vi "get bolt check tags.vi"(11 "PLC boolean read Tags":T3={"AT glass position"={"Tag Name"="", "Network Path"="", "use opc"=FALSE, "DataSocket Reference"={"CWDSLib._DCWDataSocket"=refnum, "CWDSLib._DCWData"=refnum, "OnDataUpdated"=0, "OnStatusUpdated"=0}}, "AT shade position"={"Tag Name"="", "Network Path"="", "use opc"=FALSE, "DataSocket Reference"={"CWDSLib._DCWDataSocket"=refnum, "CWDSLib._DCWData"=refnum, "OnDataUpdated"=0, "OnStatusUpdated"=0}}, "AT in glass wand lower pos"={"Tag Name"="", "Network Path"="", "use opc"=FALSE, "DataSocket Reference"={"CWDSLib._DCWDataSocket"=refnum, "CWDSLib._DCWData"=refnum, "OnDataUpdated"=0, "OnStatusUpdated"=0}}, "AT in sunshad wand lower pos"={"Tag Name"="", "Network Path"="", "use opc"=FALSE, "DataSocket Reference"={"CWDSLib._DCWDataSocket"=refnum, "CWDSLib._DCWData"=refnum, "OnDataUpdated"=0, "OnStatusUpdated"=0}}, "AT in wand home pos"={"Tag Name"="", "Network Path"="", "use opc"=FALSE, "DataSocket Reference"={"CWDSLib._DCWDataSocket"=refnum, "CWDSLib._DCWData"=refnum, "OnDataUpdated"=0, "OnStatusUpdated"=0}}, "LVDT's Extended"={"Tag Name"="", "Network Path"="", "use opc"=FALSE, "DataSocket Reference"={"CWDSLib._DCWDataSocket"=refnum, "CWDSLib._DCWData"=refnum, "OnDataUpdated"=0, "OnStatusUpdated"=0}}, "motor foam present LH"={"Tag Name"="", "Network Path"="", "use opc"=FALSE, "DataSocket Reference"={"CWDSLib._DCWDataSocket"=refnum, "CWDSLib._DCWData"=refnum, "OnDataUpdated"=0, "OnStatusUpdated"=0}}, "motor foam present RH"={"Tag Name"="", "Network Path"="", "use opc"=FALSE, "DataSocket Reference"={"CWDSLib._DCWDataSocket"=refnum, "CWDSLib._DCWData"=refnum, "OnDataUpdated"=0, "OnStatusUpdated"=0}}, "audit gap hider present LH"={"Tag Name"="", "Network Path"="", "use opc"=FALSE, "DataSocket Reference"={"CWDSLib._DCWDataSocket"=refnum, "CWDSLib._DCWData"=refnum, "OnDataUpdated"=0, "OnStatusUpdated"=0}}, "audit gap hider present RH"={"Tag Name"="", "Network Path"="", "use opc"=FALSE, "DataSocket Reference"={"CWDSLib._DCWDataSocket"=refnum, "CWDSLib._DCWData"=refnum, "OnDataUpdated"=0, "OnStatusUpdated"=0}}, "FB light block present"={"Tag Name"="", "Network Path"="", "use opc"=FALSE, "DataSocket Reference"={"CWDSLib._DCWDataSocket"=refnum, "CWDSLib._DCWData"=refnum, "OnDataUpdated"=0, "OnStatusUpdated"=0}}, "bolt check 1"={"Tag Name"="", "Network Path"="", "use opc"=FALSE, "DataSocket Reference"={"CWDSLib._DCWDataSocket"=refnum, "CWDSLib._DCWData"=refnum, "OnDataUpdated"=0, "OnStatusUpdated"=0}}, "bolt check 2"={"Tag Name"="", "Network Path"="", "use opc"=FALSE, "DataSocket Reference"={"CWDSLib._DCWDataSocket"=refnum, "CWDSLib._DCWData"=refnum, "OnDataUpdated"=0, "OnStatusUpdated"=0}}, "bolt check 3"={"Tag Name"="", "Network Path"="", "use opc"=FALSE, "DataSocket Reference"={"CWDSLib._DCWDataSocket"=refnum, "CWDSLib._DCWData"=refnum, "OnDataUpdated"=0, "OnStatusUpdated"=0}}, "bolt check 4"={"Tag Name"="", "Network Path"="", "use opc"=FALSE, "DataSocket Reference"={"CWDSLib._DCWDataSocket"=refnum, "CWDSLib._DCWData"=refnum, "OnDataUpdated"=0, "OnStatusUpdated"=0}}, "bolt check 5"={"Tag Name"="", "Network Path"="", "use opc"=FALSE, "DataSocket Reference"={"CWDSLib._DCWDataSocket"=refnum, "CWDSLib._DCWData"=refnum, "OnDataUpdated"=0, "OnStatusUpdated"=0}}, "bolt check 6"={"Tag Name"="", "Network Path"="", "use opc"=FALSE, "DataSocket Reference"={"CWDSLib._DCWDataSocket"=refnum, "CWDSLib._DCWData"=refnum, "OnDataUpdated"=0, "OnStatusUpdated"=0}}, "bolt check 7"={"Tag Name"="", "Network Path"="", "use opc"=FALSE, "DataSocket Reference"={"CWDSLib._DCWDataSocket"=refnum, "CWDSLib._DCWData"=refnum, "OnDataUpdated"=0, "OnStatusUpdated"=0}}, "bolt check 8"={"Tag Name"="", "Network Path"="", "use opc"=FALSE, "DataSocket Reference"={"CWDSLib._DCWDataSocket"=refnum, "CWDSLib._DCWData"=refnum, "OnDataUpdated"=0, "OnStatusUpdated"=0}}, "bolt check 9"={"Tag Name"="", "Network Path"="", "use opc"=FALSE, "DataSocket Reference"={"CWDSLib._DCWDataSocket"=refnum, "CWDSLib._DCWData"=refnum, "OnDataUpdated"=0, "OnStatusUpdated"=0}}, "bolt check 10"={"Tag Name"="", "Network Path"="", "use opc"=FALSE, "DataSocket Reference"={"CWDSLib._DCWDataSocket"=refnum, "CWDSLib._DCWData"=refnum, "OnDataUpdated"=0, "OnStatusUpdated"=0}}, "bolt check 11"={"Tag Name"="", "Network Path"="", "use opc"=FALSE, "DataSocket Reference"={"CWDSLib._DCWDataSocket"=refnum, "CWDSLib._DCWData"=refnum, "OnDataUpdated"=0, "OnStatusUpdated"=0}}, "bolt check 12"={"Tag Name"="", "Network Path"="", "use opc"=FALSE, "DataSocket Reference"={"CWDSLib._DCWDataSocket"=refnum, "CWDSLib._DCWData"=refnum, "OnDataUpdated"=0, "OnStatusUpdated"=0}}, "bolt check 13"={"Tag Name"="", "Network Path"="", "use opc"=FALSE, "DataSocket Reference"={"CWDSLib._DCWDataSocket"=refnum, "CWDSLib._DCWData"=refnum, "OnDataUpdated"=0, "OnStatusUpdated"=0}}, "bolt check 14"={"Tag Name"="", "Network Path"="", "use opc"=FALSE, "DataSocket Reference"={"CWDSLib._DCWDataSocket"=refnum, "CWDSLib._DCWData"=refnum, "OnDataUpdated"=0, "OnStatusUpdated"=0}}, "bolt check 15"={"Tag Name"="", "Network Path"="", "use opc"=FALSE, "DataSocket Reference"={"CWDSLib._DCWDataSocket"=refnum, "CWDSLib._DCWData"=refnum, "OnDataUpdated"=0, "OnStatusUpdated"=0}}, "bolt check 16"={"Tag Name"="", "Network Path"="", "use opc"=FALSE, "DataSocket Reference"={"CWDSLib._DCWDataSocket"=refnum, "CWDSLib._DCWData"=refnum, "OnDataUpdated"=0, "OnStatusUpdated"=0}}, "bolt check 17"={"Tag Name"="", "Network Path"="", "use opc"=FALSE, "DataSocket Reference"={"CWDSLib._DCWDataSocket"=refnum, "CWDSLib._DCWData"=refnum, "OnDataUpdated"=0, "OnStatusUpdated"=0}}, "bolt check 18"={"Tag Name"="", "Network Path"="", "use opc"=FALSE, "DataSocket Reference"={"CWDSLib._DCWDataSocket"=refnum, "CWDSLib._DCWData"=refnum, "OnDataUpdated"=0, "OnStatusUpdated"=0}}, "bolt check 19"={"Tag Name"="", "Network Path"="", "use opc"=FALSE, "DataSocket Reference"={"CWDSLib._DCWDataSocket"=refnum, "CWDSLib._DCWData"=refnum, "OnDataUpdated"=0, "OnStatusUpdated"=0}}, "bolt check 20"={"Tag Name"="", "Network Path"="", "use opc"=FALSE, "DataSocket Reference"={"CWDSLib._DCWDataSocket"=refnum, "CWDSLib._DCWData"=refnum, "OnDataUpdated"=0, "OnStatusUpdated"=0}}, "bolt check 21"={"Tag Name"="", "Network Path"="", "use opc"=FALSE, "DataSocket Reference"={"CWDSLib._DCWDataSocket"=refnum, "CWDSLib._DCWData"=refnum, "OnDataUpdated"=0, "OnStatusUpdated"=0}}, "start"={"Tag Name"="S060.PXI.Signals.PlltData.SN", "Network Path"="172.15.51.1,1,0", "use opc"=FALSE, "DataSocket Reference"={"CWDSLib._DCWDataSocket"=refnum, "CWDSLib._DCWData"=refnum, "OnDataUpdated"=0, "OnStatusUpdated"=0}}, "abort"={"Tag Name"="S060.PXI.Signals.PlltData.SN", "Network Path"="172.15.51.1,1,0", "use opc"=FALSE, "DataSocket Reference"={"CWDSLib._DCWDataSocket"=refnum, "CWDSLib._DCWData"=refnum, "OnDataUpdated"=0, "OnStatusUpdated"=0}}, "LVDT's Retracted"={"Tag Name"="S060.PXI.Signals.PlltData.SN", "Network Path"="172.15.51.1,1,0", "use opc"=FALSE, "DataSocket Reference"={"CWDSLib._DCWDataSocket"=refnum, "CWDSLib._DCWData"=refnum, "OnDataUpdated"=0, "OnStatusUpdated"=0}}, "manual barcode print"={"Tag Name"="S060.PXI.Signals.PlltData.SN", "Network Path"="172.15.51.1,1,0", "use opc"=FALSE, "DataSocket Reference"={"CWDSLib._DCWDataSocket"=refnum, "CWDSLib._DCWData"=refnum, "OnDataUpdated"=0, "OnStatusUpdated"=0}}, "ss servo at open"={"Tag Name"="S060.PXI.Signals.PlltData.SN", "Network Path"="172.15.51.1,1,0", "use opc"=FALSE, "DataSocket Reference"={"CWDSLib._DCWDataSocket"=refnum, "CWDSLib._DCWData"=refnum, "OnDataUpdated"=0, "OnStatusUpdated"=0}}, "ss servo at close"={"Tag Name"="S060.PXI.Signals.PlltData.SN", "Network Path"="172.15.51.1,1,0", "use opc"=FALSE, "DataSocket Reference"={"CWDSLib._DCWDataSocket"=refnum, "CWDSLib._DCWData"=refnum, "OnDataUpdated"=0, "OnStatusUpdated"=0}}, "ss servo opening"={"Tag Name"="S060.PXI.Signals.PlltData.SN", "Network Path"="172.15.51.1,1,0", "use opc"=FALSE, "DataSocket Reference"={"CWDSLib._DCWDataSocket"=refnum, "CWDSLib._DCWData"=refnum, "OnDataUpdated"=0, "OnStatusUpdated"=0}}, "ss servo closing"={"Tag Name"="S060.PXI.Signals.PlltData.SN", "Network Path"="172.15.51.1,1,0", "use opc"=FALSE, "DataSocket Reference"={"CWDSLib._DCWDataSocket"=refnum, "CWDSLib._DCWData"=refnum, "OnDataUpdated"=0, "OnStatusUpdated"=0}}, "control slide at home"={"Tag Name"="S060.PXI.Signals.PlltData.SN", "Network Path"="172.15.51.1,1,0", "use opc"=FALSE, "DataSocket Reference"={"CWDSLib._DCWDataSocket"=refnum, "CWDSLib._DCWData"=refnum, "OnDataUpdated"=0, "OnStatusUpdated"=0}}, "control slide left good"={"Tag Name"="S060.PXI.Signals.PlltData.SN", "Network Path"="172.15.51.1,1,0", "use opc"=FALSE, "DataSocket Reference"={"CWDSLib._DCWDataSocket"=refnum, "CWDSLib._DCWData"=refnum, "OnDataUpdated"=0, "OnStatusUpdated"=0}}, "control slide left over stroke"={"Tag Name"="S060.PXI.Signals.PlltData.SN", "Network Path"="172.15.51.1,1,0", "use opc"=FALSE, "DataSocket Reference"={"CWDSLib._DCWDataSocket"=refnum, "CWDSLib._DCWData"=refnum, "OnDataUpdated"=0, "OnStatusUpdated"=0}}, "control slide right good"={"Tag Name"="S060.PXI.Signals.PlltData.SN", "Network Path"="172.15.51.1,1,0", "use opc"=FALSE, "DataSocket Reference"={"CWDSLib._DCWDataSocket"=refnum, "CWDSLib._DCWData"=refnum, "OnDataUpdated"=0, "OnStatusUpdated"=0}}, "control slide right over stroke"={"Tag Name"="S060.PXI.Signals.PlltData.SN", "Network Path"="172.15.51.1,1,0", "use opc"=FALSE, "DataSocket Reference"={"CWDSLib._DCWDataSocket"=refnum, "CWDSLib._DCWData"=refnum, "OnDataUpdated"=0, "OnStatusUpdated"=0}}, "wind deflector high speed pos"={"Tag Name"="S060.PXI.Signals.PlltData.SN", "Network Path"="172.15.51.1,1,0", "use opc"=FALSE, "DataSocket Reference"={"CWDSLib._DCWDataSocket"=refnum, "CWDSLib._DCWData"=refnum, "OnDataUpdated"=0, "OnStatusUpdated"=0}}, "wind deflector low speed pos"={"Tag Name"="S060.PXI.Signals.PlltData.SN", "Network Path"="172.15.51.1,1,0", "use opc"=FALSE, "DataSocket Reference"={"CWDSLib._DCWDataSocket"=refnum, "CWDSLib._DCWData"=refnum, "OnDataUpdated"=0, "OnStatusUpdated"=0}}, "AT VentPMACatHome"={"Tag Name"="S060.PXI.Signals.PlltData.SN", "Network Path"="172.15.51.1,1,0", "use opc"=FALSE, "DataSocket Reference"={"CWDSLib._DCWDataSocket"=refnum, "CWDSLib._DCWData"=refnum, "OnDataUpdated"=0, "OnStatusUpdated"=0}}, "AT VentPMACisExtend"={"Tag Name"="S060.PXI.Signals.PlltData.SN", "Network Path"="172.15.51.1,1,0", "use opc"=FALSE, "DataSocket Reference"={"CWDSLib._DCWDataSocket"=refnum, "CWDSLib._DCWData"=refnum, "OnDataUpdated"=0, "OnStatusUpdated"=0}}, "SS Barcode Scanner Bypassed"={"Tag Name"="S060.PXI.Signals.PlltData.SN", "Network Path"="172.15.51.1,1,0", "use opc"=FALSE, "DataSocket Reference"={"CWDSLib._DCWDataSocket"=refnum, "CWDSLib._DCWData"=refnum, "OnDataUpdated"=0, "OnStatusUpdated"=0}}, "Check Frame Barcode"={"Tag Name"="S060.PXI.Signals.PlltData.SN", "Network Path"="172.15.51.1,1,0", "use opc"=FALSE, "DataSocket Reference"={"CWDSLib._DCWDataSocket"=refnum, "CWDSLib._DCWData"=refnum, "OnDataUpdated"=0, "OnStatusUpdated"=0}}, "iGPS Pass 0"={"Tag Name"="S060.PXI.Signals.PlltData.SN", "Network Path"="172.15.51.1,1,0", "use opc"=FALSE, "DataSocket Reference"={"CWDSLib._DCWDataSocket"=refnum, "CWDSLib._DCWData"=refnum, "OnDataUpdated"=0, "OnStatusUpdated"=0}}, "iGPS Pass 1"={"Tag Name"="S060.PXI.Signals.PlltData.SN", "Network Path"="172.15.51.1,1,0", "use opc"=FALSE, "DataSocket Reference"={"CWDSLib._DCWDataSocket"=refnum, "CWDSLib._DCWData"=refnum, "OnDataUpdated"=0, "OnStatusUpdated"=0}}, "iGPS Pass 2"={"Tag Name"="S060.PXI.Signals.PlltData.SN", "Network Path"="172.15.51.1,1,0", "use opc"=FALSE, "DataSocket Reference"={"CWDSLib._DCWDataSocket"=refnum, "CWDSLib._DCWData"=refnum, "OnDataUpdated"=0, "OnStatusUpdated"=0}}, "iGPS Pass 3"={"Tag Name"="S060.PXI.Signals.PlltData.SN", "Network Path"="172.15.51.1,1,0", "use opc"=FALSE, "DataSocket Reference"={"CWDSLib._DCWDataSocket"=refnum, "CWDSLib._DCWData"=refnum, "OnDataUpdated"=0, "OnStatusUpdated"=0}}, "iGPS Pass 4"={"Tag Name"="S060.PXI.Signals.PlltData.SN", "Network Path"="172.15.51.1,1,0", "use opc"=FALSE, "DataSocket Reference"={"CWDSLib._DCWDataSocket"=refnum, "CWDSLib._DCWData"=refnum, "OnDataUpdated"=0, "OnStatusUpdated"=0}}, "iGPS Pass 5"={"Tag Name"="S060.PXI.Signals.PlltData.SN", "Network Path"="172.15.51.1,1,0", "use opc"=FALSE, "DataSocket Reference"={"CWDSLib._DCWDataSocket"=refnum, "CWDSLib._DCWData"=refnum, "OnDataUpdated"=0, "OnStatusUpdated"=0}}, "iGPS Pass 6"={"Tag Name"="S060.PXI.Signals.PlltData.SN", "Network Path"="172.15.51.1,1,0", "use opc"=FALSE, "DataSocket Reference"={"CWDSLib._DCWDataSocket"=refnum, "CWDSLib._DCWData"=refnum, "OnDataUpdated"=0, "OnStatusUpdated"=0}}, "iGPS Pass 7"={"Tag Name"="S060.PXI.Signals.PlltData.SN", "Network Path"="172.15.51.1,1,0", "use opc"=FALSE, "DataSocket Reference"={"CWDSLib._DCWDataSocket"=refnum, "CWDSLib._DCWData"=refnum, "OnDataUpdated"=0, "OnStatusUpdated"=0}}, "iGPS Pass 8"={"Tag Name"="S060.PXI.Signals.PlltData.SN", "Network Path"="172.15.51.1,1,0", "use opc"=FALSE, "DataSocket Reference"={"CWDSLib._DCWDataSocket"=refnum, "CWDSLib._DCWData"=refnum, "OnDataUpdated"=0, "OnStatusUpdated"=0}}, "iGPS Pass 9"={"Tag Name"="S060.PXI.Signals.PlltData.SN", "Network Path"="172.15.51.1,1,0", "use opc"=FALSE, "DataSocket Reference"={"CWDSLib._DCWDataSocket"=refnum, "CWDSLib._DCWData"=refnum, "OnDataUpdated"=0, "OnStatusUpdated"=0}}, "Z LVDTs Extended"={"Tag Name"="S060.PXI.Signals.PlltData.SN", "Network Path"="172.15.51.1,1,0", "use opc"=FALSE, "DataSocket Reference"={"CWDSLib._DCWDataSocket"=refnum, "CWDSLib._DCWData"=refnum, "OnDataUpdated"=0, "OnStatusUpdated"=0}}, "NVH Operator Pass"={"Tag Name"="S060.PXI.Signals.PlltData.SN", "Network Path"="172.15.51.1,1,0", "use opc"=FALSE, "DataSocket Reference"={"CWDSLib._DCWDataSocket"=refnum, "CWDSLib._DCWData"=refnum, "OnDataUpdated"=0, "OnStatusUpdated"=0}}, "NVH Operator Fail"={"Tag Name"="S060.PXI.Signals.PlltData.SN", "Network Path"="172.15.51.1,1,0", "use opc"=FALSE, "DataSocket Reference"={"CWDSLib._DCWDataSocket"=refnum, "CWDSLib._DCWData"=refnum, "OnDataUpdated"=0, "OnStatusUpdated"=0}}, "NVH Operator Express Glass Open"={"Tag Name"="S060.PXI.Signals.PlltData.SN", "Network Path"="172.15.51.1,1,0", "use opc"=FALSE, "DataSocket Reference"={"CWDSLib._DCWDataSocket"=refnum, "CWDSLib._DCWData"=refnum, "OnDataUpdated"=0, "OnStatusUpdated"=0}}, "NVH Operator Express Glass Close"={"Tag Name"="S060.PXI.Signals.PlltData.SN", "Network Path"="172.15.51.1,1,0", "use opc"=FALSE, "DataSocket Reference"={"CWDSLib._DCWDataSocket"=refnum, "CWDSLib._DCWData"=refnum, "OnDataUpdated"=0, "OnStatusUpdated"=0}}, "NVH Operator Express Rollo Open01"={"Tag Name"="S060.PXI.Signals.PlltData.SN", "Network Path"="172.15.51.1,1,0", "use opc"=FALSE, "DataSocket Reference"={"CWDSLib._DCWDataSocket"=refnum, "CWDSLib._DCWData"=refnum, "OnDataUpdated"=0, "OnStatusUpdated"=0}}, "NVH Operator Express Rollo Close01"={"Tag Name"="S060.PXI.Signals.PlltData.SN", "Network Path"="172.15.51.1,1,0", "use opc"=FALSE, "DataSocket Reference"={"CWDSLib._DCWDataSocket"=refnum, "CWDSLib._DCWData"=refnum, "OnDataUpdated"=0, "OnStatusUpdated"=0}}, "NVH Operator Express Rollo Open02"={"Tag Name"="S060.PXI.Signals.PlltData.SN", "Network Path"="172.15.51.1,1,0", "use opc"=FALSE, "DataSocket Reference"={"CWDSLib._DCWDataSocket"=refnum, "CWDSLib._DCWData"=refnum, "OnDataUpdated"=0, "OnStatusUpdated"=0}}, "NVH Operator Express Rollo Close02"={"Tag Name"="S060.PXI.Signals.PlltData.SN", "Network Path"="172.15.51.1,1,0", "use opc"=FALSE, "DataSocket Reference"={"CWDSLib._DCWDataSocket"=refnum, "CWDSLib._DCWData"=refnum, "OnDataUpdated"=0, "OnStatusUpdated"=0}}, "NVH Operator Vent Open Noise"={"Tag Name"="S060.PXI.Signals.PlltData.SN", "Network Path"="172.15.51.1,1,0", "use opc"=FALSE, "DataSocket Reference"={"CWDSLib._DCWDataSocket"=refnum, "CWDSLib._DCWData"=refnum, "OnDataUpdated"=0, "OnStatusUpdated"=0}}, "NVH Operator Vent Close Noise"={"Tag Name"="S060.PXI.Signals.PlltData.SN", "Network Path"="172.15.51.1,1,0", "use opc"=FALSE, "DataSocket Reference"={"CWDSLib._DCWDataSocket"=refnum, "CWDSLib._DCWData"=refnum, "OnDataUpdated"=0, "OnStatusUpdated"=0}}, "NVH Operator Sunshade Open Noise"={"Tag Name"="S060.PXI.Signals.PlltData.SN", "Network Path"="172.15.51.1,1,0", "use opc"=FALSE, "DataSocket Reference"={"CWDSLib._DCWDataSocket"=refnum, "CWDSLib._DCWData"=refnum, "OnDataUpdated"=0, "OnStatusUpdated"=0}}, "NVH Operator Sunshade Close Noise"={"Tag Name"="S060.PXI.Signals.PlltData.SN", "Network Path"="172.15.51.1,1,0", "use opc"=FALSE, "DataSocket Reference"={"CWDSLib._DCWDataSocket"=refnum, "CWDSLib._DCWData"=refnum, "OnDataUpdated"=0, "OnStatusUpdated"=0}}, "NVH Operator Glass Open Noise"={"Tag Name"="S060.PXI.Signals.PlltData.SN", "Network Path"="172.15.51.1,1,0", "use opc"=FALSE, "DataSocket Reference"={"CWDSLib._DCWDataSocket"=refnum, "CWDSLib._DCWData"=refnum, "OnDataUpdated"=0, "OnStatusUpdated"=0}}, "NVH Operator Glass Close Noise"={"Tag Name"="S060.PXI.Signals.PlltData.SN", "Network Path"="172.15.51.1,1,0", "use opc"=FALSE, "DataSocket Reference"={"CWDSLib._DCWDataSocket"=refnum, "CWDSLib._DCWData"=refnum, "OnDataUpdated"=0, "OnStatusUpdated"=0}}, "NVH Operator Finish"={"Tag Name"="S060.PXI.Signals.PlltData.SN", "Network Path"="172.15.51.1,1,0", "use opc"=FALSE, "DataSocket Reference"={"CWDSLib._DCWDataSocket"=refnum, "CWDSLib._DCWData"=refnum, "OnDataUpdated"=0, "OnStatusUpdated"=0}}, "NVH Operator Check"={"Tag Name"="S060.PXI.Signals.PlltData.SN", "Network Path"="172.15.51.1,1,0", "use opc"=FALSE, "DataSocket Reference"={"CWDSLib._DCWDataSocket"=refnum, "CWDSLib._DCWData"=refnum, "OnDataUpdated"=0, "OnStatusUpdated"=0}}, "AT shade 02 position"={"Tag Name"="S060.PXI.Signals.PlltData.SN", "Network Path"="172.15.51.1,1,0", "use opc"=FALSE, "DataSocket Reference"={"CWDSLib._DCWDataSocket"=refnum, "CWDSLib._DCWData"=refnum, "OnDataUpdated"=0, "OnStatusUpdated"=0}}, "AT in sunshad 02 wand up pos"={"Tag Name"="S060.PXI.Signals.PlltData.SN", "Network Path"="172.15.51.1,1,0", "use opc"=FALSE, "DataSocket Reference"={"CWDSLib._DCWDataSocket"=refnum, "CWDSLib._DCWData"=refnum, "OnDataUpdated"=0, "OnStatusUpdated"=0}}, "AT in wand 02 home pos"={"Tag Name"="S060.PXI.Signals.PlltData.SN", "Network Path"="172.15.51.1,1,0", "use opc"=FALSE, "DataSocket Reference"={"CWDSLib._DCWDataSocket"=refnum, "CWDSLib._DCWData"=refnum, "OnDataUpdated"=0, "OnStatusUpdated"=0}}, "windproof position"={"Tag Name"="S060.PXI.Signals.PlltData.SN", "Network Path"="172.15.51.1,1,0", "use opc"=FALSE, "DataSocket Reference"={"CWDSLib._DCWDataSocket"=refnum, "CWDSLib._DCWData"=refnum, "OnDataUpdated"=0, "OnStatusUpdated"=0}}, "NVH Operator Express Glass vent Open"={"Tag Name"="S060.PXI.Signals.PlltData.SN", "Network Path"="172.15.51.1,1,0", "use opc"=FALSE, "DataSocket Reference"={"CWDSLib._DCWDataSocket"=refnum, "CWDSLib._DCWData"=refnum, "OnDataUpdated"=0, "OnStatusUpdated"=0}}, "NVH Operator Express Glass Vent Close"={"Tag Name"="S060.PXI.Signals.PlltData.SN", "Network Path"="172.15.51.1,1,0", "use opc"=FALSE, "DataSocket Reference"={"CWDSLib._DCWDataSocket"=refnum, "CWDSLib._DCWData"=refnum, "OnDataUpdated"=0, "OnStatusUpdated"=0}}, "NVH Operator Re-do"={"Tag Name"="S060.PXI.Signals.PlltData.SN", "Network Path"="172.15.51.1,1,0", "use opc"=FALSE, "DataSocket Reference"={"CWDSLib._DCWDataSocket"=refnum, "CWDSLib._DCWData"=refnum, "OnDataUpdated"=0, "OnStatusUpdated"=0}}, "AT at vent ATS test pos"={"Tag Name"="S060.PXI.Signals.PlltData.SN", "Network Path"="172.15.51.1,1,0", "use opc"=FALSE, "DataSocket Reference"={"CWDSLib._DCWDataSocket"=refnum, "CWDSLib._DCWData"=refnum, "OnDataUpdated"=0, "OnStatusUpdated"=0}}, "AT at vent ATS Home pos"={"Tag Name"="S060.PXI.Signals.PlltData.SN", "Network Path"="172.15.51.1,1,0", "use opc"=FALSE, "DataSocket Reference"={"CWDSLib._DCWDataSocket"=refnum, "CWDSLib._DCWData"=refnum, "OnDataUpdated"=0, "OnStatusUpdated"=0}}, "Start Adjust LVDT"={"Tag Name"="S060.PXI.Signals.PlltData.SN", "Network Path"="172.15.51.1,1,0", "use opc"=FALSE, "DataSocket Reference"={"CWDSLib._DCWDataSocket"=refnum, "CWDSLib._DCWData"=refnum, "OnDataUpdated"=0, "OnStatusUpdated"=0}}, "Finish Adjust LVDT"={"Tag Name"="S060.PXI.Signals.PlltData.SN", "Network Path"="172.15.51.1,1,0", "use opc"=FALSE, "DataSocket Reference"={"CWDSLib._DCWDataSocket"=refnum, "CWDSLib._DCWData"=refnum, "OnDataUpdated"=0, "OnStatusUpdated"=0}}} {"Finish Adjust LVDT"."DataSocket Reference"."OnStatusUpdated" format="%.0x"; "Finish Adjust LVDT"."DataSocket Reference"."OnDataUpdated" format="%.0x"; "Start Adjust LVDT"."DataSocket Reference"."OnStatusUpdated" format="%.0x"; "Start Adjust LVDT"."DataSocket Reference"."OnDataUpdated" format="%.0x"; "AT at vent ATS Home pos"."DataSocket Reference"."OnStatusUpdated" format="%.0x"; "AT at vent ATS Home pos"."DataSocket Reference"."OnDataUpdated" format="%.0x"; "AT at vent ATS test pos"."DataSocket Reference"."OnStatusUpdated" format="%.0x"; "AT at vent ATS test pos"."DataSocket Reference"."OnDataUpdated" format="%.0x"; "NVH Operator Re-do"."DataSocket Reference"."OnStatusUpdated" format="%.0x"; "NVH Operator Re-do"."DataSocket Reference"."OnDataUpdated" format="%.0x"; "NVH Operator Express Glass Vent Close"."DataSocket Reference"."OnStatusUpdated" format="%.0x"; "NVH Operator Express Glass Vent Close"."DataSocket Reference"."OnDataUpdated" format="%.0x"; "NVH Operator Express Glass vent Open"."DataSocket Reference"."OnStatusUpdated" format="%.0x"; "NVH Operator Express Glass vent Open"."DataSocket Reference"."OnDataUpdated" format="%.0x"; "windproof position"."DataSocket Reference"."OnStatusUpdated" format="%.0x"; "windproof position"."DataSocket Reference"."OnDataUpdated" format="%.0x"; "AT in wand 02 home pos"."DataSocket Reference"."OnStatusUpdated" format="%.0x"; "AT in wand 02 home pos"."DataSocket Reference"."OnDataUpdated" format="%.0x"; "AT in sunshad 02 wand up pos"."DataSocket Reference"."OnStatusUpdated" format="%.0x"; "AT in sunshad 02 wand up pos"."DataSocket Reference"."OnDataUpdated" format="%.0x"; "AT shade 02 position"."DataSocket Reference"."OnStatusUpdated" format="%.0x"; "AT shade 02 position"."DataSocket Reference"."OnDataUpdated" format="%.0x"; "NVH Operator Check"."DataSocket Reference"."OnStatusUpdated" format="%.0x"; "NVH Operator Check"."DataSocket Reference"."OnDataUpdated" format="%.0x"; "NVH Operator Finish"."DataSocket Reference"."OnStatusUpdated" format="%.0x"; "NVH Operator Finish"."DataSocket Reference"."OnDataUpdated" format="%.0x"; "NVH Operator Glass Close Noise"."DataSocket Reference"."OnStatusUpdated" format="%.0x"; "NVH Operator Glass Close Noise"."DataSocket Reference"."OnDataUpdated" format="%.0x"; "NVH Operator Glass Open Noise"."DataSocket Reference"."OnStatusUpdated" format="%.0x"; "NVH Operator Glass Open Noise"."DataSocket Reference"."OnDataUpdated" format="%.0x"; "NVH Operator Sunshade Close Noise"."DataSocket Reference"."OnStatusUpdated" format="%.0x"; "NVH Operator Sunshade Close Noise"."DataSocket Reference"."OnDataUpdated" format="%.0x"; "NVH Operator Sunshade Open Noise"."DataSocket Reference"."OnStatusUpdated" format="%.0x"; "NVH Operator Sunshade Open Noise"."DataSocket Reference"."OnDataUpdated" format="%.0x"; "NVH Operator Vent Close Noise"."DataSocket Reference"."OnStatusUpdated" format="%.0x"; "NVH Operator Vent Close Noise"."DataSocket Reference"."OnDataUpdated" format="%.0x"; "NVH Operator Vent Open Noise"."DataSocket Reference"."OnStatusUpdated" format="%.0x"; "NVH Operator Vent Open Noise"."DataSocket Reference"."OnDataUpdated" format="%.0x"; "NVH Operator Express Rollo Close02"."DataSocket Reference"."OnStatusUpdated" format="%.0x"; "NVH Operator Express Rollo Close02"."DataSocket Reference"."OnDataUpdated" format="%.0x"; "NVH Operator Express Rollo Open02"."DataSocket Reference"."OnStatusUpdated" format="%.0x"; "NVH Operator Express Rollo Open02"."DataSocket Reference"."OnDataUpdated" format="%.0x"; "NVH Operator Express Rollo Close01"."DataSocket Reference"."OnStatusUpdated" format="%.0x"; "NVH Operator Express Rollo Close01"."DataSocket Reference"."OnDataUpdated" format="%.0x"; "NVH Operator Express Rollo Open01"."DataSocket Reference"."OnStatusUpdated" format="%.0x"; "NVH Operator Express Rollo Open01"."DataSocket Reference"."OnDataUpdated" format="%.0x"; "NVH Operator Express Glass Close"."DataSocket Reference"."OnStatusUpdated" format="%.0x"; "NVH Operator Express Glass Close"."DataSocket Reference"."OnDataUpdated" format="%.0x"; "NVH Operator Express Glass Open"."DataSocket Reference"."OnStatusUpdated" format="%.0x"; "NVH Operator Express Glass Open"."DataSocket Reference"."OnDataUpdated" format="%.0x"; "NVH Operator Fail"."DataSocket Reference"."OnStatusUpdated" format="%.0x"; "NVH Operator Fail"."DataSocket Reference"."OnDataUpdated" format="%.0x"; "NVH Operator Pass"."DataSocket Reference"."OnStatusUpdated" format="%.0x"; "NVH Operator Pass"."DataSocket Reference"."OnDataUpdated" format="%.0x"; "Z LVDTs Extended"."DataSocket Reference"."OnStatusUpdated" format="%.0x"; "Z LVDTs Extended"."DataSocket Reference"."OnDataUpdated" format="%.0x"; "iGPS Pass 9"."DataSocket Reference"."OnStatusUpdated" format="%.0x"; "iGPS Pass 9"."DataSocket Reference"."OnDataUpdated" format="%.0x"; "iGPS Pass 8"."DataSocket Reference"."OnStatusUpdated" format="%.0x"; "iGPS Pass 8"."DataSocket Reference"."OnDataUpdated" format="%.0x"; "iGPS Pass 7"."DataSocket Reference"."OnStatusUpdated" format="%.0x"; "iGPS Pass 7"."DataSocket Reference"."OnDataUpdated" format="%.0x"; "iGPS Pass 6"."DataSocket Reference"."OnStatusUpdated" format="%.0x"; "iGPS Pass 6"."DataSocket Reference"."OnDataUpdated" format="%.0x"; "iGPS Pass 5"."DataSocket Reference"."OnStatusUpdated" format="%.0x"; "iGPS Pass 5"."DataSocket Reference"."OnDataUpdated" format="%.0x"; "iGPS Pass 4"."DataSocket Reference"."OnStatusUpdated" format="%.0x"; "iGPS Pass 4"."DataSocket Reference"."OnDataUpdated" format="%.0x"; "iGPS Pass 3"."DataSocket Reference"."OnStatusUpdated" format="%.0x"; "iGPS Pass 3"."DataSocket Reference"."OnDataUpdated" format="%.0x"; "iGPS Pass 2"."DataSocket Reference"."OnStatusUpdated" format="%.0x"; "iGPS Pass 2"."DataSocket Reference"."OnDataUpdated" format="%.0x"; "iGPS Pass 1"."DataSocket Reference"."OnStatusUpdated" format="%.0x"; "iGPS Pass 1"."DataSocket Reference"."OnDataUpdated" format="%.0x"; "iGPS Pass 0"."DataSocket Reference"."OnStatusUpdated" format="%.0x"; "iGPS Pass 0"."DataSocket Reference"."OnDataUpdated" format="%.0x"; "Check Frame Barcode"."DataSocket Reference"."OnStatusUpdated" format="%.0x"; "Check Frame Barcode"."DataSocket Reference"."OnDataUpdated" format="%.0x"; "SS Barcode Scanner Bypassed"."DataSocket Reference"."OnStatusUpdated" format="%.0x"; "SS Barcode Scanner Bypassed"."DataSocket Reference"."OnDataUpdated" format="%.0x"; "AT VentPMACisExtend"."DataSocket Reference"."OnStatusUpdated" format="%.0x"; "AT VentPMACisExtend"."DataSocket Reference"."OnDataUpdated" format="%.0x"; "AT VentPMACatHome"."DataSocket Reference"."OnStatusUpdated" format="%.0x"; "AT VentPMACatHome"."DataSocket Reference"."OnDataUpdated" format="%.0x"; "wind deflector low speed pos"."DataSocket Reference"."OnStatusUpdated" format="%.0x"; "wind deflector low speed pos"."DataSocket Reference"."OnDataUpdated" format="%.0x"; "wind deflector high speed pos"."DataSocket Reference"."OnStatusUpdated" format="%.0x"; "wind deflector high speed pos"."DataSocket Reference"."OnDataUpdated" format="%.0x"; "control slide right over stroke"."DataSocket Reference"."OnStatusUpdated" format="%.0x"; "control slide right over stroke"."DataSocket Reference"."OnDataUpdated" format="%.0x"; "control slide right good"."DataSocket Reference"."OnStatusUpdated" format="%.0x"; "control slide right good"."DataSocket Reference"."OnDataUpdated" format="%.0x"; "control slide left over stroke"."DataSocket Reference"."OnStatusUpdated" format="%.0x"; "control slide left over stroke"."DataSocket Reference"."OnDataUpdated" format="%.0x"; "control slide left good"."DataSocket Reference"."OnStatusUpdated" format="%.0x"; "control slide left good"."DataSocket Reference"."OnDataUpdated" format="%.0x"; "control slide at home"."DataSocket Reference"."OnStatusUpdated" format="%.0x"; "control slide at home"."DataSocket Reference"."OnDataUpdated" format="%.0x"; "ss servo closing"."DataSocket Reference"."OnStatusUpdated" format="%.0x"; "ss servo closing"."DataSocket Reference"."OnDataUpdated" format="%.0x"; "ss servo opening"."DataSocket Reference"."OnStatusUpdated" format="%.0x"; "ss servo opening"."DataSocket Reference"."OnDataUpdated" format="%.0x"; "ss servo at close"."DataSocket Reference"."OnStatusUpdated" format="%.0x"; "ss servo at close"."DataSocket Reference"."OnDataUpdated" format="%.0x"; "ss servo at open"."DataSocket Reference"."OnStatusUpdated" format="%.0x"; "ss servo at open"."DataSocket Reference"."OnDataUpdated" format="%.0x"; "manual barcode print"."DataSocket Reference"."OnStatusUpdated" format="%.0x"; "manual barcode print"."DataSocket Reference"."OnDataUpdated" format="%.0x"; "LVDT's Retracted"."DataSocket Reference"."OnStatusUpdated" format="%.0x"; "LVDT's Retracted"."DataSocket Reference"."OnDataUpdated" format="%.0x"; "abort"."DataSocket Reference"."OnStatusUpdated" format="%.0x"; "abort"."DataSocket Reference"."OnDataUpdated" format="%.0x"; "start"."DataSocket Reference"."OnStatusUpdated" format="%.0x"; "start"."DataSocket Reference"."OnDataUpdated" format="%.0x"; "bolt check 21"."DataSocket Reference"."OnStatusUpdated" format="%.0x"; "bolt check 21"."DataSocket Reference"."OnDataUpdated" format="%.0x"; "bolt check 20"."DataSocket Reference"."OnStatusUpdated" format="%.0x"; "bolt check 20"."DataSocket Reference"."OnDataUpdated" format="%.0x"; "bolt check 19"."DataSocket Reference"."OnStatusUpdated" format="%.0x"; "bolt check 19"."DataSocket Reference"."OnDataUpdated" format="%.0x"; "bolt check 18"."DataSocket Reference"."OnStatusUpdated" format="%.0x"; "bolt check 18"."DataSocket Reference"."OnDataUpdated" format="%.0x"; "bolt check 17"."DataSocket Reference"."OnStatusUpdated" format="%.0x"; "bolt check 17"."DataSocket Reference"."OnDataUpdated" format="%.0x"; "bolt check 16"."DataSocket Reference"."OnStatusUpdated" format="%.0x"; "bolt check 16"."DataSocket Reference"."OnDataUpdated" format="%.0x"; "bolt check 15"."DataSocket Reference"."OnStatusUpdated" format="%.0x"; "bolt check 15"."DataSocket Reference"."OnDataUpdated" format="%.0x"; "bolt check 14"."DataSocket Reference"."OnStatusUpdated" format="%.0x"; "bolt check 14"."DataSocket Reference"."OnDataUpdated" format="%.0x"; "bolt check 13"."DataSocket Reference"."OnStatusUpdated" format="%.0x"; "bolt check 13"."DataSocket Reference"."OnDataUpdated" format="%.0x"; "bolt check 12"."DataSocket Reference"."OnStatusUpdated" format="%.0x"; "bolt check 12"."DataSocket Reference"."OnDataUpdated" format="%.0x"; "bolt check 11"."DataSocket Reference"."OnStatusUpdated" format="%.0x"; "bolt check 11"."DataSocket Reference"."OnDataUpdated" format="%.0x"; "bolt check 10"."DataSocket Reference"."OnStatusUpdated" format="%.0x"; "bolt check 10"."DataSocket Reference"."OnDataUpdated" format="%.0x"; "bolt check 9"."DataSocket Reference"."OnStatusUpdated" format="%.0x"; "bolt check 9"."DataSocket Reference"."OnDataUpdated" format="%.0x"; "bolt check 8"."DataSocket Reference"."OnStatusUpdated" format="%.0x"; "bolt check 8"."DataSocket Reference"."OnDataUpdated" format="%.0x"; "bolt check 7"."DataSocket Reference"."OnStatusUpdated" format="%.0x"; "bolt check 7"."DataSocket Reference"."OnDataUpdated" format="%.0x"; "bolt check 6"."DataSocket Reference"."OnStatusUpdated" format="%.0x"; "bolt check 6"."DataSocket Reference"."OnDataUpdated" format="%.0x"; "bolt check 5"."DataSocket Reference"."OnStatusUpdated" format="%.0x"; "bolt check 5"."DataSocket Reference"."OnDataUpdated" format="%.0x"; "bolt check 4"."DataSocket Reference"."OnStatusUpdated" format="%.0x"; "bolt check 4"."DataSocket Reference"."OnDataUpdated" format="%.0x"; "bolt check 3"."DataSocket Reference"."OnStatusUpdated" format="%.0x"; "bolt check 3"."DataSocket Reference"."OnDataUpdated" format="%.0x"; "bolt check 2"."DataSocket Reference"."OnStatusUpdated" format="%.0x"; "bolt check 2"."DataSocket Reference"."OnDataUpdated" format="%.0x"; "bolt check 1"."DataSocket Reference"."OnStatusUpdated" format="%.0x"; "bolt check 1"."DataSocket Reference"."OnDataUpdated" format="%.0x"; "FB light block present"."DataSocket Reference"."OnStatusUpdated" format="%.0x"; "FB light block present"."DataSocket Reference"."OnDataUpdated" format="%.0x"; "audit gap hider present RH"."DataSocket Reference"."OnStatusUpdated" format="%.0x"; "audit gap hider present RH"."DataSocket Reference"."OnDataUpdated" format="%.0x"; "audit gap hider present LH"."DataSocket Reference"."OnStatusUpdated" format="%.0x"; "audit gap hider present LH"."DataSocket Reference"."OnDataUpdated" format="%.0x"; "motor foam present RH"."DataSocket Reference"."OnStatusUpdated" format="%.0x"; "motor foam present RH"."DataSocket Reference"."OnDataUpdated" format="%.0x"; "motor foam present LH"."DataSocket Reference"."OnStatusUpdated" format="%.0x"; "motor foam present LH"."DataSocket Reference"."OnDataUpdated" format="%.0x"; "LVDT's Extended"."DataSocket Reference"."OnStatusUpdated" format="%.0x"; "LVDT's Extended"."DataSocket Reference"."OnDataUpdated" format="%.0x"; "AT in wand home pos"."DataSocket Reference"."OnStatusUpdated" format="%.0x"; "AT in wand home pos"."DataSocket Reference"."OnDataUpdated" format="%.0x"; "AT in sunshad wand lower pos"."DataSocket Reference"."OnStatusUpdated" format="%.0x"; "AT in sunshad wand lower pos"."DataSocket Reference"."OnDataUpdated" format="%.0x"; "AT in glass wand lower pos"."DataSocket Reference"."OnStatusUpdated" format="%.0x"; "AT in glass wand lower pos"."DataSocket Reference"."OnDataUpdated" format="%.0x"; "AT shade position"."DataSocket Reference"."OnStatusUpdated" format="%.0x"; "AT shade position"."DataSocket Reference"."OnDataUpdated" format="%.0x"; "AT glass position"."DataSocket Reference"."OnStatusUpdated" format="%.0x"; "AT glass position"."DataSocket Reference"."OnDataUpdated" format="%.0x"}) -> (3 "bolt check tags":T1[](array[typedef]) {"DataSocket Reference"."OnStatusUpdated" format="%.0x"; "DataSocket Reference"."OnDataUpdated" format="%.0x"})   [LabVIEW 2018]
uses:
  02.Type Def's/station plc read boolean tags.ctl
  05.UserVI's/type defs/plc path and tag.ctl
  <vilib>/Platform/dataskt.llb/DataSocket Reference Type.ctl
panel:
  # "start/abort only used by barcode instance, since there are discrete signals for this in the other stations."
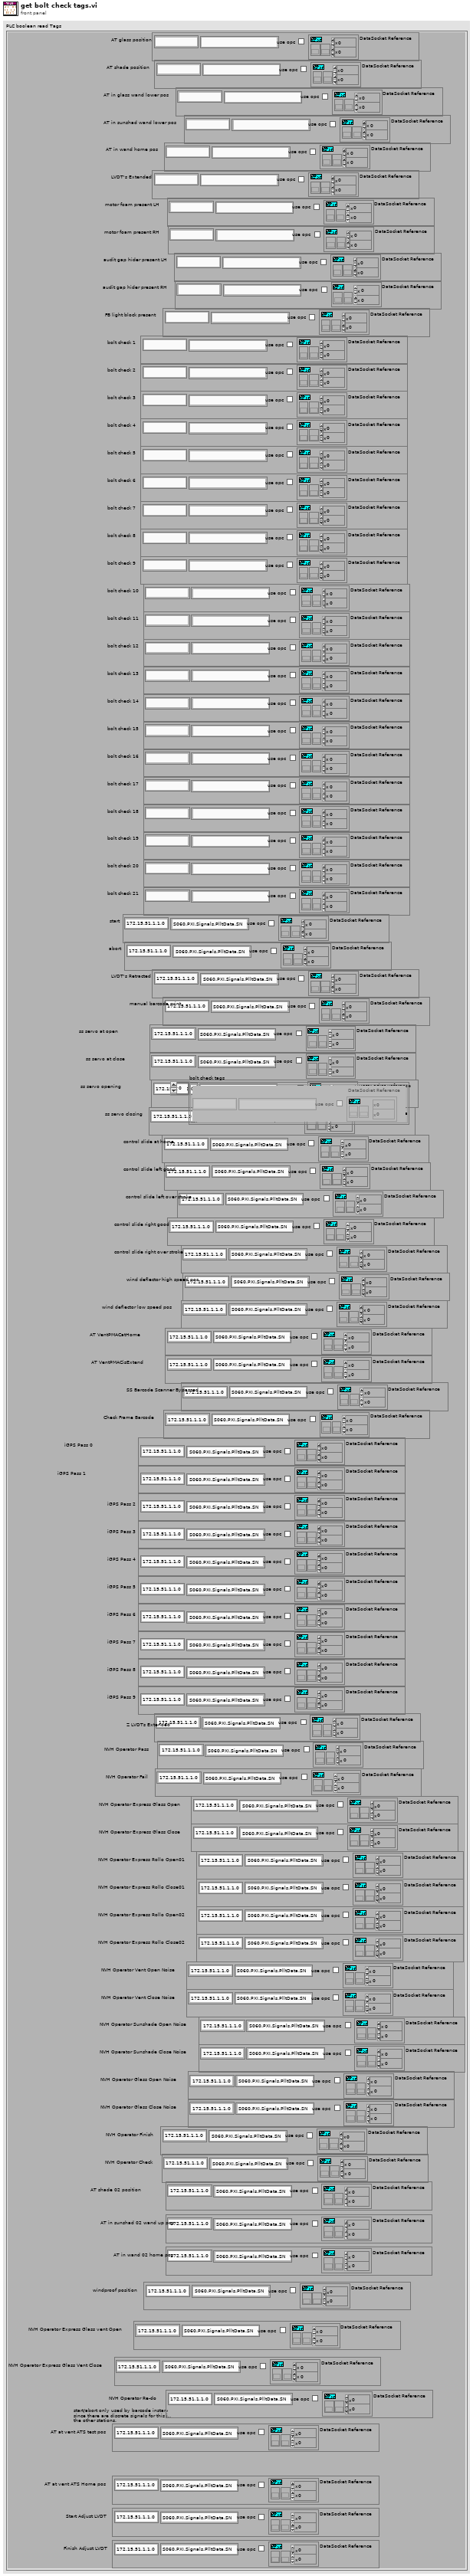
[diagram p1: front panel]
types:
  T1 = typedef "plc path and tag.ctl" = cluster{"Tag Name":string, "Network Path":string, "use opc":bool, "DataSocket Reference":T2}
  T2 = typedef "DataSocket Reference Type.ctl" = cluster{"CWDSLib._DCWDataSocket":refnum<k7>, "CWDSLib._DCWData":refnum<k7>, "OnDataUpdated":u32, "OnStatusUpdated":u32}
  T3 = typedef "station plc read boolean tags.ctl" = cluster{"AT glass position":T1, "AT shade position":T1, "AT in glass wand lower pos":T1, "AT in sunshad wand lower pos":T1, "AT in wand home pos":T1, "LVDT's Extended":T1, "motor foam present LH":T1, "motor foam present RH":T1, "audit gap hider present LH":T1, "audit gap hider present RH":T1, "FB light block present":T1, "bolt check 1":T1, "bolt check 2":T1, "bolt check 3":T1, "bolt check 4":T1, "bolt check 5":T1, "bolt check 6":T1, "bolt check 7":T1, "bolt check 8":T1, "bolt check 9":T1, "bolt check 10":T1, "bolt check 11":T1, "bolt check 12":T1, "bolt check 13":T1, "bolt check 14":T1, "bolt check 15":T1, "bolt check 16":T1, "bolt check 17":T1, "bolt check 18":T1, "bolt check 19":T1, "bolt check 20":T1, "bolt check 21":T1, "start":T1, "abort":T1, "LVDT's Retracted":T1, "manual barcode print":T1, "ss servo at open":T1, "ss servo at close":T1, "ss servo opening":T1, "ss servo closing":T1, "control slide at home":T1, "control slide left good":T1, "control slide left over stroke":T1, "control slide right good":T1, "control slide right over stroke":T1, "wind deflector high speed pos":T1, "wind deflector low speed pos":T1, "AT VentPMACatHome":T1, "AT VentPMACisExtend":T1, "SS Barcode Scanner Bypassed":T1, "Check Frame Barcode":T1, "iGPS Pass 0":T1, "iGPS Pass 1":T1, "iGPS Pass 2":T1, "iGPS Pass 3":T1, "iGPS Pass 4":T1, "iGPS Pass 5":T1, "iGPS Pass 6":T1, "iGPS Pass 7":T1, "iGPS Pass 8":T1, "iGPS Pass 9":T1, "Z LVDTs Extended":T1, "NVH Operator Pass":T1, "NVH Operator Fail":T1, "NVH Operator Express Glass Open":T1, "NVH Operator Express Glass Close":T1, "NVH Operator Express Rollo Open01":T1, "NVH Operator Express Rollo Close01":T1, "NVH Operator Express Rollo Open02":T1, "NVH Operator Express Rollo Close02":T1, "NVH Operator Vent Open Noise":T1, "NVH Operator Vent Close Noise":T1, "NVH Operator Sunshade Open Noise":T1, "NVH Operator Sunshade Close Noise":T1, "NVH Operator Glass Open Noise":T1, "NVH Operator Glass Close Noise":T1, "NVH Operator Finish":T1, "NVH Operator Check":T1, "AT shade 02 position":T1, "AT in sunshad 02 wand up pos":T1, "AT in wand 02 home pos":T1, "windproof position":T1, "NVH Operator Express Glass vent Open":T1, "NVH Operator Express Glass Vent Close":T1, "NVH Operator Re-do":T1, "AT at vent ATS test pos":T1, "AT at vent ATS Home pos":T1, "Start Adjust LVDT":T1, "Finish Adjust LVDT":T1}
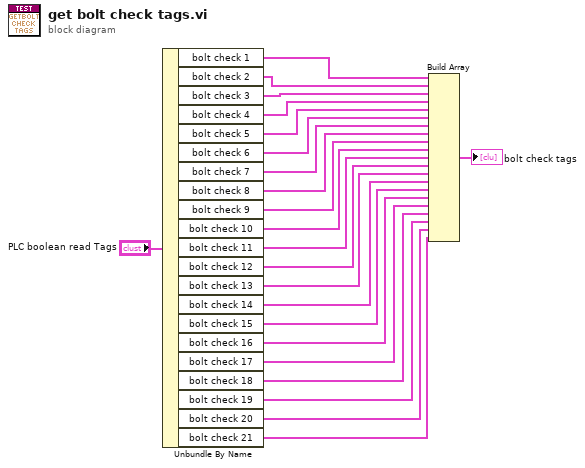
[diagram p0: block diagram]
diagram:
  n1 = Unbundle By Name("PLC boolean read Tags") -> ("bolt check 1"=w23:T1, "bolt check 2"=w22:T1, "bolt check 3"=w20:T1, "bolt check 4"=w19:T1, "bolt check 5"=w18:T1, "bolt check 6"=w17:T1, "bolt check 7"=w16:T1, "bolt check 8"=w15:T1, "bolt check 9"=w14:T1, "bolt check 10"=w13:T1, "bolt check 11"=w12:T1, "bolt check 12"=w11:T1, "bolt check 13"=w10:T1, "bolt check 14"=w9:T1, "bolt check 15"=w8:T1, "bolt check 16"=w7:T1, "bolt check 17"=w6:T1, "bolt check 18"=w5:T1, "bolt check 19"=w4:T1, "bolt check 20"=w3:T1, "bolt check 21"=w2:T1)
  n2 = Build Array(w23, w22, w20, w19, w18, w17, w16, w15, w14, w13, w12, w11, w10, w9, w8, w7, w6, w5, w4, w3, w2) -> (→"bolt check tags":T1[])
